vi "Feed Controller.vi"(8 "error in":errorcluster) -> ()   [LabVIEW 2019]
doc: "This VI executes continuously carrying out the current operation and responding to updates or new operations. It will often contain the timing or control code that is difficult to place directly in TeleOp. This VI generally opens all sensors and motors and isolates the rest of the robot code from knowing how the operations are carried out."
uses:
  <vilib>/Rock Robotics/WPI/Framework/Completion Status.ctl
  Feed Setpoints.ctl
  Feed Operations.ctl
  <vilib>/Rock Robotics/SystemInterfaces/i2clib/i2c_bus.ctl
  <vilib>/Rock Robotics/WPI/ThirdParty/Phoenix-LabVIEW/Motor Controller/Controls/CTRE_Phoenix_MotorControl_ControlMode.ctl
  <vilib>/Rock Robotics/Network Tables/NT Write Numeric Array.vi
  <vilib>/Rock Robotics/Network Tables/NT Write Number.vi
  Framework/Robot Global Data.vi
  <vilib>/Rock Robotics/Network Tables/NT Write Variant.vi
  <vilib>/Rock Robotics/Network Tables/NT Write Boolean.vi
panel:
  out "Confidence Output":dbl
  in  "Confidence Threshold":dbl
  in  "Interactive Values":T1
  out "Current\nCmd":string
  in  "Buttons":cluster{"Execute Cmd":bool, "Abort Cmd":bool}
  out "Command Timing":cluster{"Start Time (ms)":u32, "Iterations":i32}
  out "Status":T3
  # "Tip: It may be helpful to observe inputs and sensor values.\nYou may also want to display tuning or debugging controls."
  # "Interactive Command: You may fill in the settings for a command\nand schedule it with the Execute button. You can observe and abort\nany command while fine tuning the code for the controller."
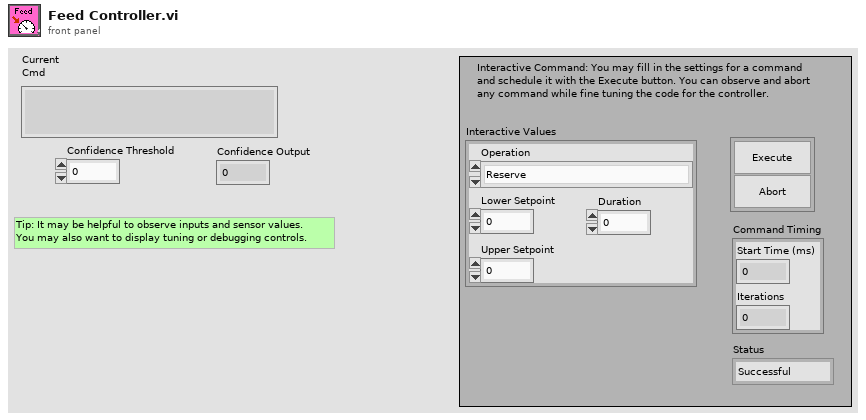
[diagram p1: front panel]
types:
  T1 = typedef "Feed Setpoints.ctl" = cluster{"Operation":T2, "Lower Setpoint":dbl, "Upper Setpoint":dbl, "Duration":dbl}
  T2 = typedef "Feed Operations.ctl" = enum16{"Reserve", "Read Current", "Immediate", "Feed For Time"}
  T3 = typedef "Completion Status.ctl" = enum16{"Successful", "Aborted", "Incomplete"}
  T4 = typedef "i2c_bus.ctl" = enum16{"I2C On-Board", "I2C MXP", "Invalid"}
  T5 = typedef "WPI_MotorControlDeviceRef.ctl" = cluster{"DeviceStatus":errorcluster, "Type":T6, "PWM":cluster{"PWM Channel":T7, "DeadBand":T8}, "CAN":cluster{"Device Number":u8, "SetOutput VI Ref":variant, "GetOutput VI Ref":variant, "Enable VI Ref":variant, "Disable VI Ref":variant, "Data":variant}, "Invert":bool, "DIO PWM":cluster{"PWM \"Enable\" Channel":T7, "DIOChannel":T9, "PWM Rate":dbl}}
  T6 = typedef "WPI_MotorControlType.ctl" = enum16{"PWM", "CAN", "DIO PWM"}
  T7 = typedef "FPGA_DIOPWMChannel.ctl" = enum8{"PWM 0", "PWM 1", "PWM 2", "PWM 3", "PWM 4", "PWM 5", "PWM 6", "PWM 7", "PWM 8", "PWM 9", "PWM MXP 0", "PWM MXP 1", "PWM MXP 2", "PWM MXP 3", "PWM MXP 4", "PWM MXP 5", "PWM MXP 6", "PWM MXP 7", "PWM MXP 8", "PWM MXP 9", "Invalid"}
  T8 = typedef "WPI_PWMDeadband.ctl" = cluster{"Name":string, "maxPositivePwm":i32, "minPositivePwm":i32, "centerPwm":i32, "maxNegativePwm":i32, "minNegativePwm":i32, "angularRange":u16}
  T9 = typedef "FPGA_DIOChannel.ctl" = enum8{"DIO 0", "DIO 1", "DIO 2", "DIO 3", "DIO 4", "DIO 5", "DIO 6", "DIO 7", "DIO 8", "DIO 9", "DIO MXP 0", "DIO MXP 1", "DIO MXP 2", "DIO MXP 3", "DIO MXP 4", "DIO MXP 5", "DIO MXP 6", "DIO MXP 7", "DIO MXP 8", "DIO MXP 9", "DIO MXP 10", "DIO MXP 11", "DIO MXP 12", "DIO MXP 13", "DIO MXP 14", "DIO MXP 15", "SPI Port CS1", "SPI Port CS2", "SPI Port CS3", "SPI Port MISO", "SPI Port MOSI", "Invalid"}
  T10 = typedef "Color Sensor V3 DevRef.ctl" = cluster{"I2CDevRef":T11}
  T11 = typedef "WPI_I2CDevRef.ctl" = cluster{"DevStatus":errorcluster, "Device Address":u8, "Handle":i32, "I2C Bus":T4}
  T12 = typedef "Command Status Info.ctl" = cluster{"Name":string, "Status":T3, "notifier out":T13}
  T13 = typedef "Completion Notifier.ctl" = refnum<notifier>
  T14 = cluster{"Current Command":T1, "Command Timing":cluster{"Start Time (ms)":u32, "Iterations":i32}, "Command Arguments":cluster{"Command Info":T12, "Description":string, "Default Command":T1, "queue out":refnum<queue>, "Subsystem Name":string}}
  T15 = enum16{"DemandType_Neutral", "DemandType_AuxPID", "DemandType_ArbitraryFeedForward"}
  T16 = typedef "CTRE_Phoenix_MotorControl_ControlMode.ctl" = u16
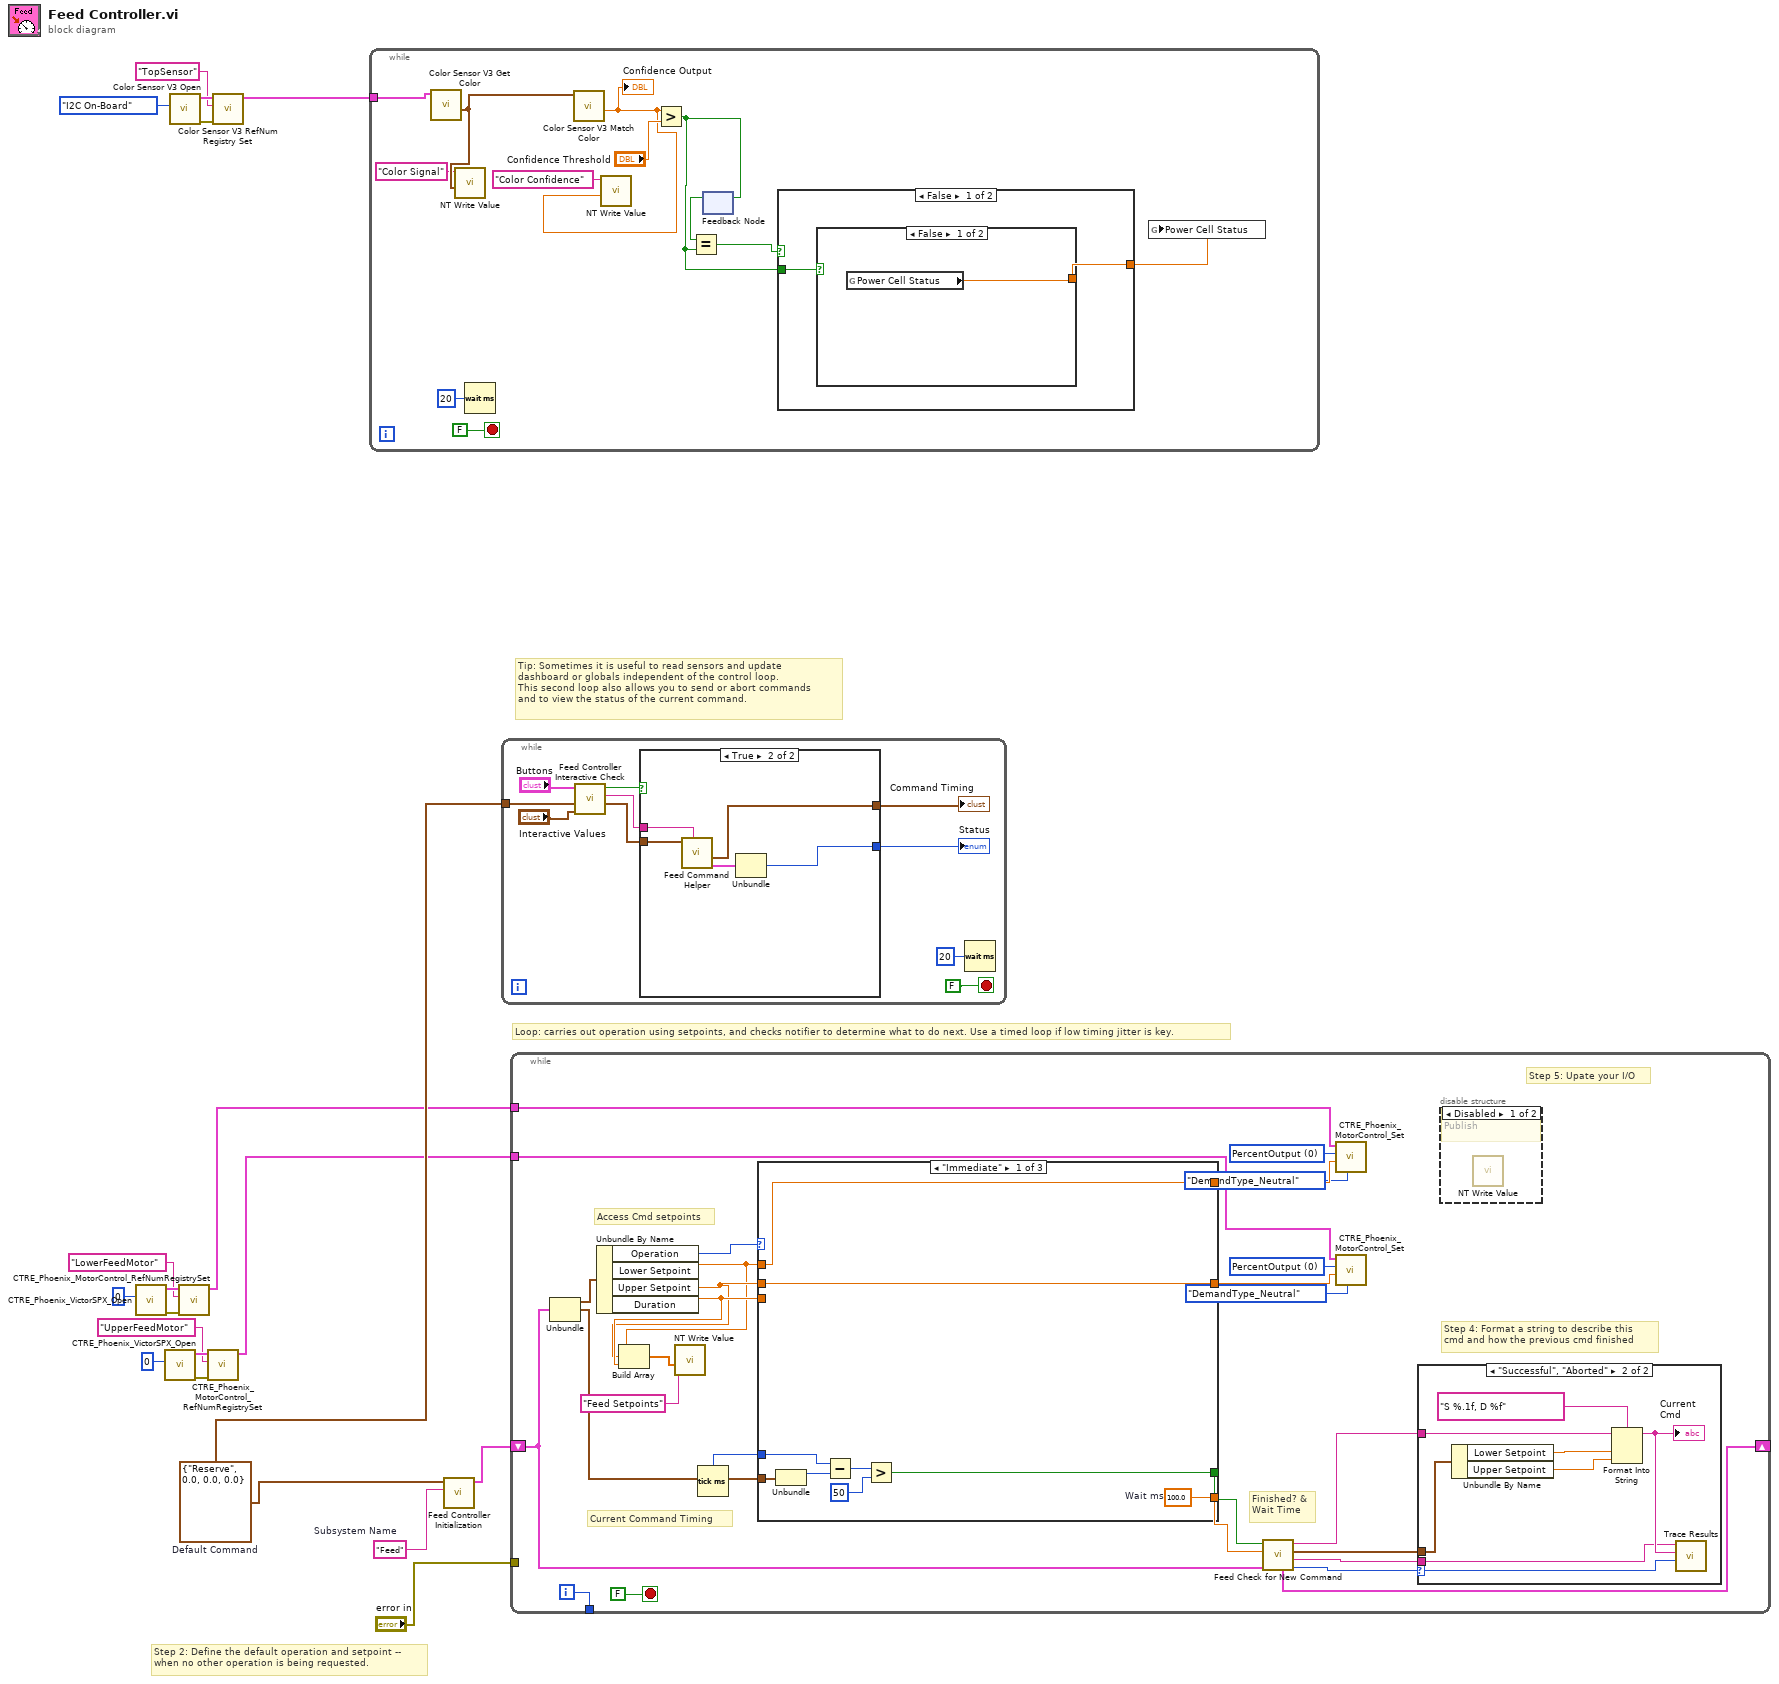
[diagram p0: block diagram]
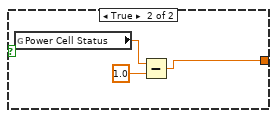
[diagram p2: hidden frame]
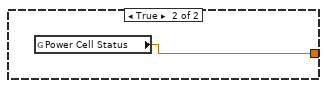
[diagram p3: hidden frame]
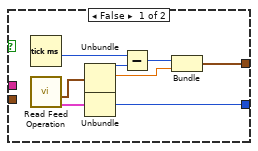
[diagram p4: hidden frame]
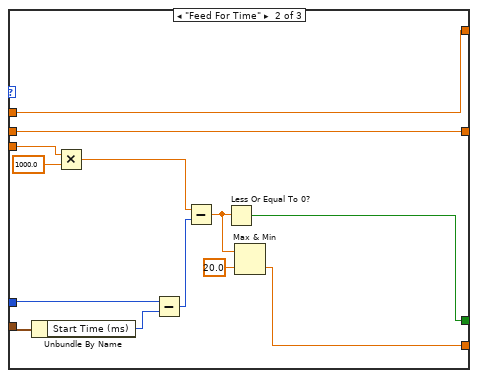
[diagram p7: hidden frame]
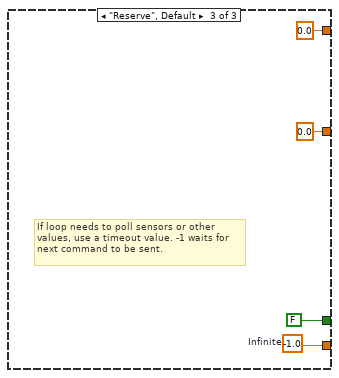
[diagram p8: hidden frame]
diagram:
  w16 = T1 {"Operation"=enum."Reserve", "Lower Setpoint"=0.0, "Upper Setpoint"=0.0, "Duration"=0.0}  # Default Command
  w17 = "Feed"  # Subsystem Name
  # "Tip: Sometimes it is useful to read sensors and update\ndashboard or globals independent of the control loop.\nThis second loop also allows you to send or abort commands\nand to view the status of the current command."
  # "Step 2: Define the default operation and setpoint --\nwhen no other operation is being requested."
  # "Loop: carries out operation using setpoints, and checks notifier to determine what to do next. Use a timed loop if low timing jitter is key."
  n1 = call <vilib>:"CTRE_Phoenix_VictorSPX_Open.vi"("Device Number"=u8 0) -> ("error out"=w15:errorcluster, "CAN Talon SRX Ref"=w14:T5)  [unwired: 9 in]
  n2 = call <vilib>:"CTRE_Phoenix_VictorSPX_Open.vi"("Device Number"=u8 0) -> ("error out"=w12:errorcluster, "CAN Talon SRX Ref"=w11:T5)  [unwired: 9 in]
  n3 = call <vilib>:"Color Sensor V3 Open.vi"("I2C Bus"=i2c_bus."I2C On-Board") -> ("error out"=w4:errorcluster, "ColorSensorDevRef"=w3:T10)  [unwired: 9 in]
  n4 = call <vilib>:"CTRE_Phoenix_MotorControl_RefNumRegistrySet.vi"("error in (no error)"=w15, "refnum name"="LowerFeedMotor", "PhoenixMotorControlDevRef"=w14) -> ("PhoenixMotorControlDevRef"=w7:T5)  [unwired: 7 in, 1 out]
  n5 = call <vilib>:"CTRE_Phoenix_MotorControl_RefNumRegistrySet.vi"("error in (no error)"=w12, "refnum name"="UpperFeedMotor", "PhoenixMotorControlDevRef"=w11) -> ("PhoenixMotorControlDevRef"=w8:T5)  [unwired: 7 in, 1 out]
  n6 = call <vilib>:"Color Sensor V3 RefNum Registry Set.vi"("error in (no error)"=w4, "refnum name"="TopSensor", "ColorSensorDevRef"=w3) -> ("ColorSensorDevRef out"=w1:T10)  [unwired: 7 in, 1 out]
  n7 = while {
    tunnel: w1 -> [w24]
    stop <- FALSE stop-if-true
    n8 = call <vilib>:"Color Sensor V3 Get Color.vi"("ColorSensorDevRef"=w24) -> ("Normalized Color"=w23:cluster{"R":dbl, "G":dbl, "B":dbl})  [unwired: 7 in, 3 out]
    n9 = call-poly <vilib>:"NT Write Value.vi"("Variant"=w23, "Name"="Color Signal") -> ()  [unwired: 9 in, 1 out]
    n10 = Wait (ms)(milliseconds to wait=u32 20) -> ()  [unwired: 1 out]
    n11 = call <vilib>:"Color Sensor V3 Match Color.vi"("Measured Color"=w23) -> ("Confidence"=w20:dbl)  [unwired: 8 in, 2 out]
    "Confidence Output" <- w20
    n12 = call-poly <vilib>:"NT Write Value.vi"("Numeric"=w20, "Name"="Color Confidence") -> ()  [unwired: 9 in, 1 out]
    n13 = Greater?(x=w20, y="Confidence Threshold") -> (0:w25:bool)
    n14 = feedback-in #1(w25) -> ()
    n15 = feedback #1() -> (w27:bool)  [unwired: 1 in]
    n16 = Equal?(x=w27, y=w25) -> (x = y?=w26:bool)
    n17 = case shown="False" w26 {
      tunnel: [w33 w38] -> w30
      tunnel: w25 -> [w32 _]
      frame False {
        n18 = case shown="False" w32 {
          tunnel: [w34 w35] -> w33
          frame False {
            n19 = global read "Robot Global Data.vi" "Power Cell Status"() -> (w34:dbl)
          }
          frame True {
            n20 = global read "Robot Global Data.vi" "Power Cell Status"() -> (w37:dbl)
            n21 = Subtract(x=w37, y=1.0) -> (x-y=w35:dbl)
          }
        }
      }
      frame True {
        n22 = global read "Robot Global Data.vi" "Power Cell Status"() -> (w38:dbl)
      }
    }
    n23 = global write "Robot Global Data.vi" "Power Cell Status"(w30) -> ()
  }
  n24 = call "Feed Controller Initialization.vi"("Subsystem Name"=w17, "Default Command"=w16) -> ("Current Command"=w18:T14)  [unwired: 9 in]
  n25 = while {
    tunnel: w16 -> [w45]
    stop <- FALSE stop-if-true
    n26 = call "Feed Controller Interactive Check.vi"("Interactive Command in"="Interactive Values", "Default Command"=w45, "Buttons"="Buttons") -> ("Interactive Command out"=w42:T1, "Trace String"=w43:string, "Schedule"=w44:bool)  [unwired: 6 in]
    n27 = case shown="True" w44 {
      tunnel: [w56 w61] -> w41
      tunnel: w42 -> [_ w59]
      tunnel: [w52 w57] -> w40
      tunnel: w43 -> [_ w60]
      frame False {
        n28 = Tick Count (ms)() -> (millisecond timer value=w51:u32)
        n29 = call "Read Feed Operation.vi"() -> ("Command Info"=w49:T12, "SubSystem Data"=w50:T1)  [unwired: 9 in, 1 out]
        n30 = Unbundle(w50) -> ("Operation"=w55:T2, "Lower Setpoint"=w53:dbl)  [unwired: 2 out]
        n31 = Unbundle(w49) -> ("Status"=w56:T3)  [unwired: 2 out]
        n32 = Subtract(x=w51, y=w55) -> (x-y=w54:u32)
        n33 = Bundle(w54, "Lower Setpoint"=w53) -> (w52:cluster{u32, "Lower Setpoint":dbl})  [unwired: 1 in]
      }
      frame True {
        n34 = call "Feed Command Helper.vi"("Description"=w60, "SubSystem Data"=w59) -> ("Command Info Out"=w58:T12, "Command Timing"=w57:cluster{"Start Time (ms)":u32, "Iterations":i32})  [unwired: 7 in, 1 out]
        n35 = Unbundle(w58) -> ("Status"=w61:T3)  [unwired: 2 out]
      }
    }
    "Status" <- w41
    "Command Timing" <- w40
    n36 = Wait (ms)(milliseconds to wait=u32 20) -> ()  [unwired: 1 out]
  }
  n37 = while {
    shift-right: [w82] -> _
    shift-left: w18 -> [w75]
    tunnel: [w87] -> _
    tunnel: "error in" -> [_]
    tunnel: w8 -> [w74]
    tunnel: w7 -> [w73]
    i -> [w87]
    stop <- FALSE stop-if-true
    w69 = T16 0 items=["PercentOutput"=0, "Position"=1, "Velocity"=2, "Current"=3, "Follower"=5, "MotionProfile"=6, "MotionMagic"=7, "MotionProfileArc"=10, "Disabled"=15] ("Control Mode")
    w70 = T16 0 items=["PercentOutput"=0, "Position"=1, "Velocity"=2, "Current"=3, "Follower"=5, "MotionProfile"=6, "MotionMagic"=7, "MotionProfileArc"=10, "Disabled"=15] ("Control Mode")
    # "Step 5: Upate your I/O"
    # "Step 4: Format a string to describe this\ncmd and how the previous cmd finished"
    # "Current Command Timing"
    # "Access Cmd setpoints"
    # "Finished? &\nWait Time"
    n38 = Unbundle(w75) -> ("Current Command"=w86:T1, "Command Timing"=w83:cluster{"Start Time (ms)":u32, "Iterations":i32})  [unwired: 1 out]
    n39 = Unbundle By Name(w86) -> ("Operation"=w85:T2, "Lower Setpoint"=w64:dbl, "Upper Setpoint"=w65:dbl, "Duration"=w66:dbl)
    n40 = Build Array(w64, w65, w66) -> (w63:dbl[])
    n41 = call-poly <vilib>:"NT Write Value.vi"("Numeric Array"=w63, "Name"="Feed Setpoints") -> ()  [unwired: 9 in, 1 out]
    n42 = Tick Count (ms)() -> (millisecond timer value=w84:u32)
    n43 = case shown="\"Immediate\"" w85 {
      tunnel: [w105 w106 w122] -> w80
      tunnel: [w99 w109 FALSE ("ignore previous (F)")] -> w81
      tunnel: w83 -> [w101 w116 _]
      tunnel: w64 -> [w97 w118 _]
      tunnel: w84 -> [w100 w114 _]
      tunnel: w65 -> [w98 w117 _]
      tunnel: [w97 w118 0.0 ("Lower Setpoint")] -> w72
      tunnel: [w98 w117 0.0 ("Upper Setpoint")] -> w71
      tunnel: w66 -> [_ w113 _]
      frame "Immediate" {
        w105 = 100.0  # Wait ms
        n44 = Unbundle(w101) -> ("Start Time (ms)"=w104:u32)  [unwired: 1 out]
        n45 = Subtract(x=w100, y=w104) -> (x-y=w103:u32)
        n46 = Greater?(x=w103, y=u8 50 ("Left Motor")) -> (0:w99:bool)
      }
      frame "Feed For Time" {
        n47 = Unbundle By Name(w116) -> ("Start Time (ms)"=w115:u32)
        n48 = Multiply(x=w113, y=1000.0) -> (x*y=w110:dbl)
        n49 = Subtract(x=w114, y=w115) -> (x-y=w111:u32)
        n50 = Subtract(x=w110, y=w111) -> (x-y=w108:dbl)
        n51 = Less Or Equal To 0?(x=w108) -> (x <= 0?=w109:bool)
        n52 = Max & Min(x=w108, y=20.0) -> (min(x,y)=w106:dbl)  [unwired: 1 out]
      }
      frame "Reserve", Default {
        w122 = -1.0  # Infinite
        # "If loop needs to poll sensors or other\nvalues, use a timeout value. -1 waits for\nnext command to be sent."
      }
    }
    n53 = call "Feed Check for New Command.vi"("Current Command"=w75, "Wait time (ms)"=w80, "Finished?"=w81) -> ("Completion"=w76:T3, "Subsystem Name"=w77:string, "Current Command"=w78:T1, "Initial Trace String"=w79:string, "NextCommand"=w82:T14)  [unwired: 4 in]
    n54 = call <vilib>:"CTRE_Phoenix_MotorControl_Set.vi"("DemandType"=T15."DemandType_Neutral", "Output"=w72, "Control Mode"=w70, "PhoenixMotorControlDevRef"=w73) -> ()  [unwired: 6 in, 2 out]
    n55 = call <vilib>:"CTRE_Phoenix_MotorControl_Set.vi"("DemandType"=T15."DemandType_Neutral", "Output"=w71, "Control Mode"=w69, "PhoenixMotorControlDevRef"=w74) -> ()  [unwired: 6 in, 2 out]
    n56 = case shown="\"Successful\", \"Aborted\"" w76 {
      selector: w76 -> [_ w96]
      tunnel: w79 -> [_ w92]
      tunnel: w78 -> [_ w93]
      tunnel: w77 -> [_ w89]
      frame "Incomplete", Default {
        # "Continuing current command"
      }
      frame "Successful", "Aborted" {
        # "Report and setup for next command"
        n57 = Unbundle By Name(w93) -> ("Lower Setpoint"=w95:dbl, "Upper Setpoint"=w90:dbl)
        n58 = Format Into String(format string="S %.1f, D %f", initial string=w92, w95, w90) -> (resulting string=w91:string)  [unwired: 1 in, 1 out]
        "Current\nCmd" <- w91
        n59 = call <vilib>:"Trace Results.vi"("Status of previous command"=w96, "Description"=w91, "Subsystem"=w89) -> ()  [unwired: 9 in]
      }
    }
    n60 = disable-structure shown="Disabled" {
      frame Disabled {
        # "Publish"
        n61 = call-poly <vilib>:"NT Write Value.vi"() -> ()  [unwired: 11 in, 1 out]
      }
      frame Enabled {
      }
    }
  }
